vi "Test Failed Method.vi"(8 "error in (no error)":errorcluster, 11 "Test Case In":refnum<class "Result Table Test.lvclass">) -> (0 "error out":errorcluster, 3 "Test Case Out":refnum<class "Result Table Test.lvclass">)   [LabVIEW 2020, in "LUnit Tests.lvlib" / "Result Table Test.lvclass"]
uses:
  Result Table Test.lvclass
  Result Table Test.lvclass/Result Table Test.ctl
  01074fa8-ee8a-411d-bc8b-fc92c4f90959.vi
  source/Framework/Helper Classes/Result Table/Result Table/Result Table.lvclass
  source/Framework/Result Types/Assertion Result/Public/TypeDefs/Status.ctl
  source/Framework/Result Types/Assertion Result/Assertion Result.lvlib
panel:
  out "Result Texts":string[](array[string])
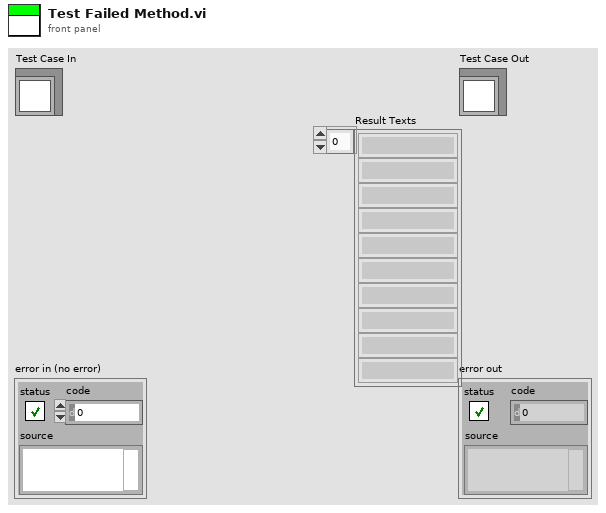
[diagram p1: front panel]
types:
  T1 = typedef "Assertion Result.lvlib/Status.ctl" = enum16{"Pass", "Fail", "Error", "Skipped", "Setup Error", "Broken", "Teardown Error"}
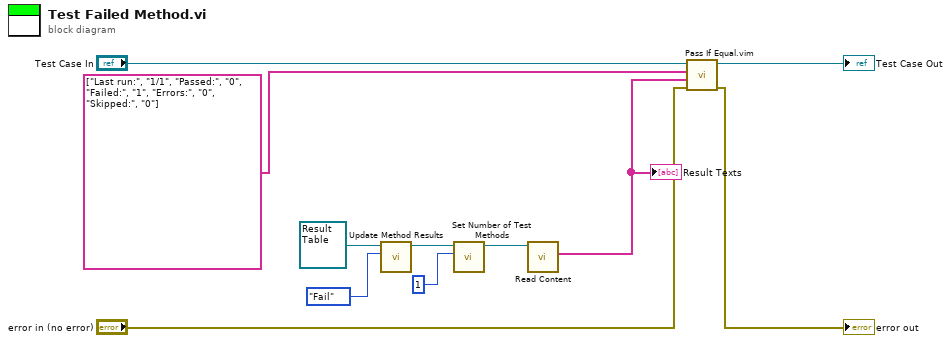
[diagram p0: block diagram]
diagram:
  n1 = call "Update Method Results.vi"("Method Result"=Status."Fail", "Result Table in"=refnum<class "Result Table.lvclass"> refnum ("Result Table.lvclass")) -> ("Result Table out"=w4:refnum<class "Result Table.lvclass">)  [unwired: 8 in, 1 out]
  n2 = call "Set Number of Test Methods.vi"("Method Count"=u32 1, "Result Table.lvclass"=w4) -> ("Result Table"=w2:refnum<class "Result Table.lvclass">)  [unwired: 8 in, 1 out]
  n3 = call "Read Content.vi"("Result Table in"=w2) -> ("Result Texts"=w7:string[])  [unwired: 8 in, 2 out]
  "Result Texts" <- w7
  n4 = call "Pass If Equal.vim"("error in (no error)"="error in (no error)", "Actual"=w7, "Expected"=string[] ["Last run:", "1/1", "Passed:", "0", "Failed:", "1", "Errors:", "0", "Skipped:", "0"], "LUnit Test Case In"="Test Case In") -> ("error out"=→"error out":errorcluster, "LUnit Test Case Out"=→"Test Case Out":refnum<class "Result Table Test.lvclass">)  [unwired: 6 in]
